vi "test Parse File Info.vi"(11 "Test Case In":refnum<class "test EDS.lvclass">) -> (0 "error out":errorcluster, 3 "Test Case Out":refnum<class "test EDS.lvclass">)   [LabVIEW 2024, in "Test EDS.lvclass"]
uses:
  test EDS.lvclass
  Core/EDS/EDS.lvclass
  <vilib>/PNR/JSONtext Object Serialization/Generic Object Serializer/Generic Object Serializer.lvclass
  <vilib>/PNR/JSONtext Object Serialization/Generic Object Serializer/Type Name Handling.ctl
  <vilib>/PNR/JSONtext Object Serialization/Generic Object Serializer/Generic Object Serializer.lvclass/Generic Object Serializer.ctl
  Core/EDS/EDS.lvclass/EDS.ctl
  <vilib>/Astemes/LUnit/Test Case.lvclass/Test Case.ctl
  e7a2ff47-5664-4bcf-a5df-3b8eb6edaa5e.vi
  4993e8ee-a06a-463a-9684-69129f64d5ce.vi
  <vilib>/PNR/JSONtext Object Serialization/Generic Object Serializer/Write Type Name Handling.vi
  <vilib>/Astemes/LUnit/Append Pass Result.vi
  <vilib>/Astemes/LUnit/Append Fail Result.vi
  <vilib>/Astemes/LUnit/Describe Comparison.vi
  4993e8ee-a06a-463a-9684-69129f64d5ce.vi/9c5d11cd-9439-4240-a1ee-d9baace9c924.vi
  <vilib>/Astemes/LUnit/Run In UI.vi
  <vilib>/Utility/error.llb/Clear Errors.vi
  <vilib>/JDP Science/JSONtext/Variant to JSON Text.vi
  <vilib>/Astemes/LUnit/Describe Variant.vi
  test EDS.lvclass/test EDS.ctl
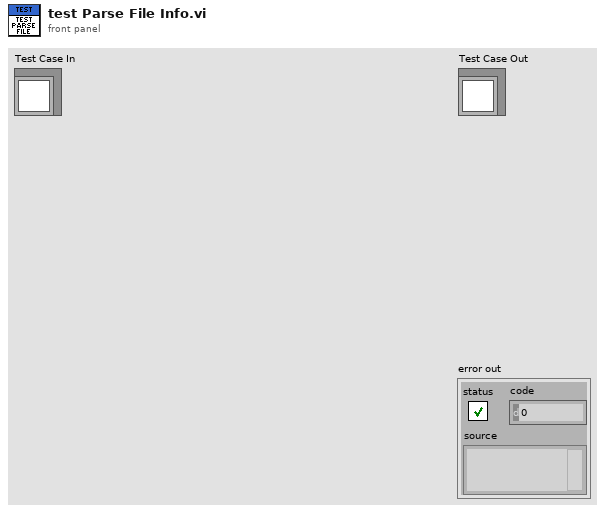
[diagram p1: front panel]
types:
  T1 = typedef "Generic Object Serializer.lvclass/Type Name Handling.ctl" = enum16{"None", "Inline"}
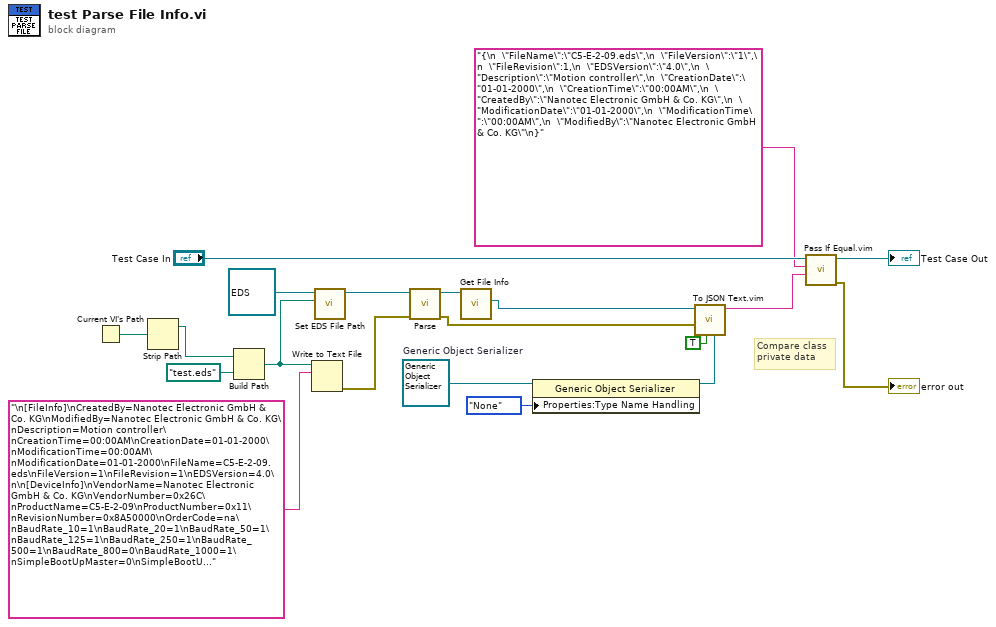
[diagram p0: block diagram]
diagram:
  w7 = refnum<class "Generic Object Serializer.lvclass"> refnum  # Generic Object Serializer
  # "Compare class\nprivate data"
  n1 = Current VI's Path() -> (path=w16:path)
  n2 = Strip Path(path=w16) -> (stripped path=w15:path)  [unwired: 1 out]
  n3 = Build Path(base path=w15, name or relative path=path "test.eds") -> (appended path=w14:path)
  n4 = Write to Text File(file (use dialog)=w14, text="\n[FileInfo]\nCreatedBy=Nanotec Electronic GmbH & Co. KG\nModifiedBy=Nanotec Electronic GmbH & Co. KG\nDescription=Motion controller\nCreationTime=00:00AM\nCreationDate=01-01-2000\nModificationTime=00:00AM\nModificationDate=01-01-2000\nFileName=C5-E-2-09.eds\nFileVersion=1\nFileRevision=1\nEDSVersion=4.0\n\n[DeviceInfo]\nVendorName=Nanotec Electronic GmbH & Co. KG\nVendorNumber=0x26C\nProductName=C5-E-2-09\nProductNumber=0x11\nRevisionNumber=0x8A50000\nOrderCode=na\nBaudRate_10=1\nBaudRate_20=1\nBaudRate_50=1\nBaudRate_125=1\nBaudRate_250=1\nBaudRate_500=1\nBaudRate_800=0\nBaudRate_1000=1\nSimpleBootUpMaster=0\nSimpleBootUpSlave=0\nGranularity=8\nDynamicChannelsSupported=0\nCompactPDO=0\nGroupMessaging=0\nNrOfRXPDO=8\nNrOfTXPDO=8\nLSS_Supported=0\n") -> (error out=w12:errorcluster)  [unwired: 2 in, 2 out]
  n5 = call "Set EDS File Path.vi"("EDS File Path"=w14, "EDS in"=refnum<class "EDS.lvclass"> refnum ("EDS.lvlib:EDS.lvclass")) -> ("EDS out"=w17:refnum<class "EDS.lvclass">)  [unwired: 9 in]
  n6 = call "Parse.vi"("error in"=w12, "EDS in"=w17) -> ("error out"=w3:errorcluster, "EDS out"=w10:refnum<class "EDS.lvclass">)  [unwired: 8 in]
  n7 = call "Get File Info.vi"("EDS in"=w10) -> ("File Info"=w1:refnum<class "File Info.lvclass">)  [unwired: 9 in, 1 out]
  n8 = property class="Generic Object Serializer"(reference=w7, "Properties:Type Name Handling"=Type_Name_Handling."None" ("Type Name Handling")) -> (reference out=w6:refnum<class "Generic Object Serializer.lvclass">)  [unwired: 1 in, 1 out]
  n9 = call "To JSON Text.vim"("LVClass Serializer"=w6, "Pretty Print?"=TRUE, "error in (no error)"=w3, "Anything"=w1) -> ("<JSON>"=w2:string)  [unwired: 6 in, 1 out]
  n10 = call "Pass If Equal.vim"("Actual"=w2, "Expected"="{\n  \"FileName\":\"C5-E-2-09.eds\",\n  \"FileVersion\":\"1\",\n  \"FileRevision\":1,\n  \"EDSVersion\":\"4.0\",\n  \"Description\":\"Motion controller\",\n  \"CreationDate\":\"01-01-2000\",\n  \"CreationTime\":\"00:00AM\",\n  \"CreatedBy\":\"Nanotec Electronic GmbH & Co. KG\",\n  \"ModificationDate\":\"01-01-2000\",\n  \"ModificationTime\":\"00:00AM\",\n  \"ModifiedBy\":\"Nanotec Electronic GmbH & Co. KG\"\n}" ("<JSON>"), "LUnit Test Case In"="Test Case In") -> ("error out"=→"error out":errorcluster, "LUnit Test Case Out"=→"Test Case Out":refnum<class "test EDS.lvclass">)  [unwired: 7 in]
